vi "Get Configuration Interface.vi"(8 "error in":errorcluster, 11 "Plugin_Controller in":refnum<class "Plugin_Controller.lvclass">) -> (0 "error out":errorcluster, 2 "Configuration Interface":refnum<class "Configuration Interface.lvclass">, 3 "Plugin_Controller out":refnum<class "Plugin_Controller.lvclass">)   [LabVIEW 2020, in "Plugin.lvlib" / "Plugin_Controller.lvclass"]
doc: "Gets the Plugin's Configuration Interface class"
uses:
  Plugin_Controller.lvclass
  builds/Libraries/LabSys Framework.lvlibp/Configurable Data Node/Configuration Interface/Configuration Interface.lvclass
  UI_Class/Plugin_UI.lvclass
  C:/SVN_LabSys/labsys_lvcode/LabSys_SourceCode/builds/Libraries/LabSys Framework.lvlibp/Configurable Data Node/Configuration Interface/Configuration Interface.lvclass
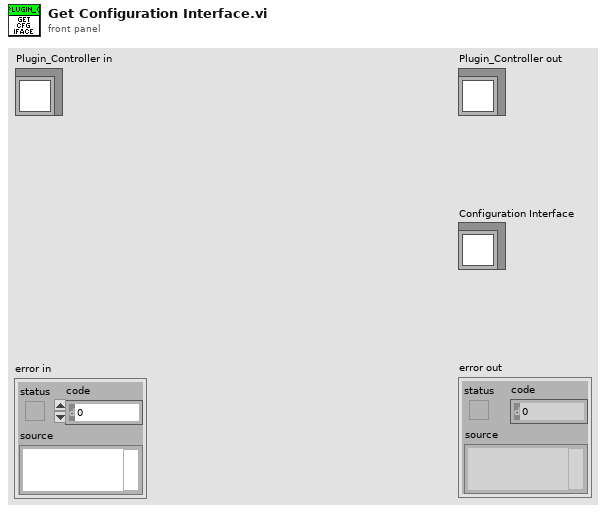
[diagram p1: front panel]
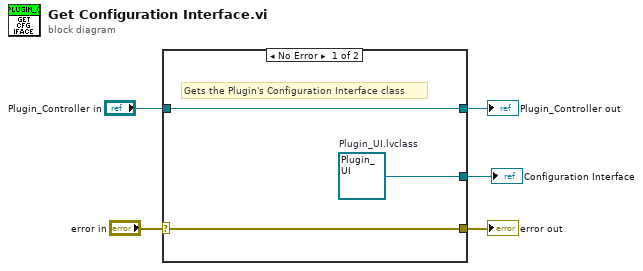
[diagram p0: block diagram]
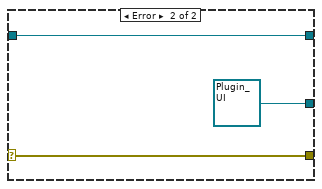
[diagram p2: hidden frame]
diagram:
  n1 = case shown="No Error" "error in" {
    selector: "error in" -> [w7 w11]
    tunnel: [w7 w11] -> w4
    tunnel: [w8 w10] -> w2
    tunnel: "Plugin_Controller in" -> [w8 w10]
    tunnel: [w6 refnum<class "Plugin_UI.lvclass"> refnum ("Plugin_UI.lvclass")] -> w1
    frame No Error {
      w6 = refnum<class "Plugin_UI.lvclass"> refnum  # Plugin_UI.lvclass
      # "Gets the Plugin's Configuration Interface class"
    }
    frame Error {
    }
  }
  "error out" <- w4
  "Plugin_Controller out" <- w2
  "Configuration Interface" <- w1
